vi "Set Batch of Controls.vi"(8 "error in (no error)":errorcluster, 9 "Indicator Values":variant[](array[variant]), 10 "Indicator Names":string[](array[string]), 11 "Rename in":refnum<class "Rename.lvclass">) -> (0 "error out":errorcluster, 3 "Rename out":refnum<class "Rename.lvclass">)   [LabVIEW 2015, in "Generic Module Library.lvlib" / "Template G_Module.lvlib" / "Rename.lvclass"]
uses:
  Rename.lvclass
  Private API/Module Control Manager/Control_Mgr_Class/Controls_Mgr.lvclass
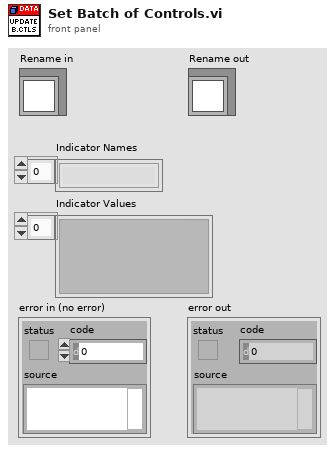
[diagram p1: front panel]
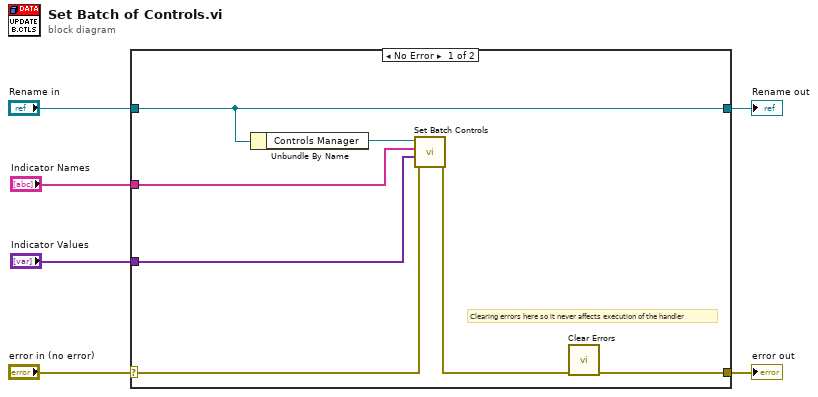
[diagram p0: block diagram]
diagram:
  n1 = case shown="No Error" "error in (no error)" {
    selector: "error in (no error)" -> [w11 w15]
    tunnel: [w7 w15] -> w5
    tunnel: [w13 w14] -> w3
    tunnel: "Rename in" -> [w13 w14]
    tunnel: "Indicator Names" -> [w8 _]
    tunnel: "Indicator Values" -> [w9 _]
    frame No Error {
      # "Clearing errors here so it never affects execution of the handler"
      n2 = Unbundle By Name(w13) -> ("Controls Manager"=w12:refnum<class "Controls_Mgr.lvclass">)
      n3 = call "Set Batch Controls.vi"("error in (no error)"=w11, "Indicator Values"=w9, "Indicator Names"=w8, "Controls_Mgr in"=w12) -> ("error out"=w10:errorcluster)  [unwired: 6 in, 1 out]
      n4 = call <vilib>:"Clear Errors.vi"("error in (no error)"=w10) -> ("error out"=w7:errorcluster)  [unwired: 5 in, 1 out]
    }
    frame Error {
    }
  }
  "error out" <- w5
  "Rename out" <- w3
